vi "Set ADB Location.vi"(8 "error in (no error)":errorcluster, 10 "adb path":path, 11 "AdbBridge in":refnum<class "Adb Bridge.lvclass">) -> (0 "error out":errorcluster, 3 "AdbBridge out":refnum<class "Adb Bridge.lvclass">)   [LabVIEW 2016, in "Adb Bridge.lvclass"]
uses:
  Adb Bridge.lvclass
  Adb Bridge.lvclass/Adb Bridge.ctl
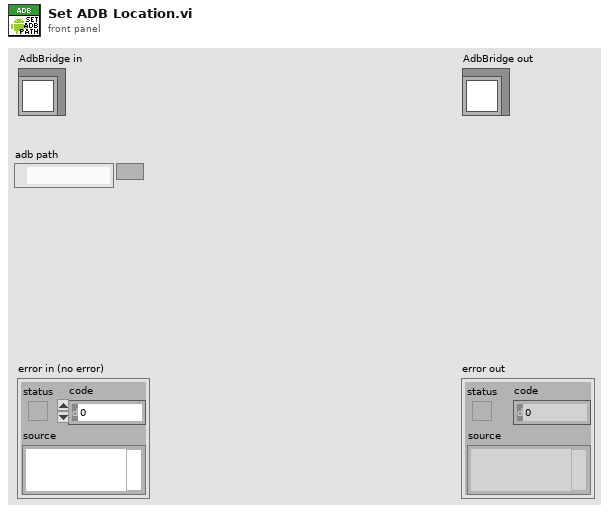
[diagram p1: front panel]
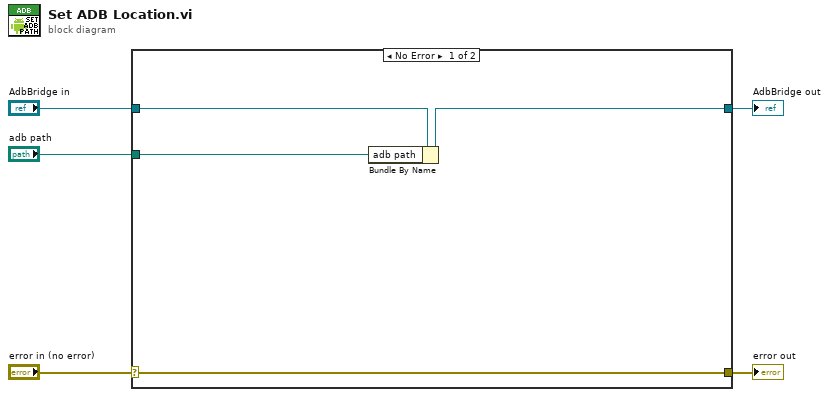
[diagram p0: block diagram]
diagram:
  n1 = case shown="No Error" "error in (no error)" {
    selector: "error in (no error)" -> [w8 w11]
    tunnel: [w8 w11] -> w4
    tunnel: [w7 w10] -> w2
    tunnel: "AdbBridge in" -> [w9 w10]
    tunnel: "adb path" -> [w6 _]
    frame No Error {
      n2 = Bundle By Name(cluster=w9, "adb path"=w6) -> (w7:refnum<class "Adb Bridge.lvclass">)
    }
    frame Error {
    }
  }
  "error out" <- w4
  "AdbBridge out" <- w2
